vi "Inhibit Bus B.vi"(8 "error in (no error)":errorcluster, 10 "Inhibit Bus B?":bool, 11 "1553 Component in":refnum<class "1553 Component.lvclass">) -> (0 "error out":errorcluster)   [LabVIEW 2020, in "BCI-1553 API.lvlib" / "1553 Component.lvclass"]
doc: "Inhibit the operation of Bus B for this component."
uses:
  1553 Component.lvclass
  1553 Component.lvclass/1553 Component.ctl
  Dependencies/FPGA Interface/FPGA Interface.lvclass
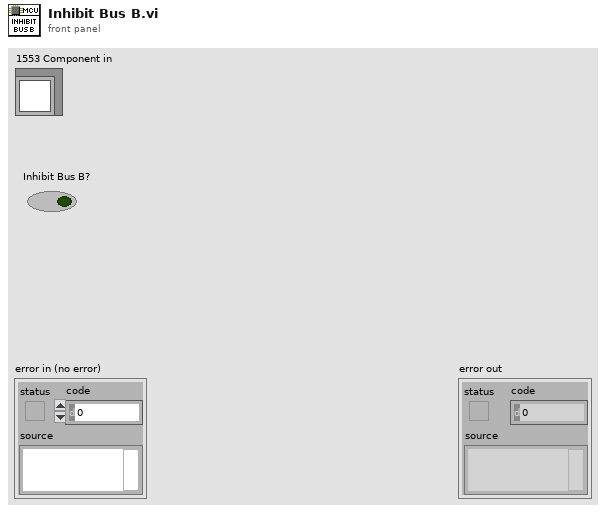
[diagram p1: front panel]
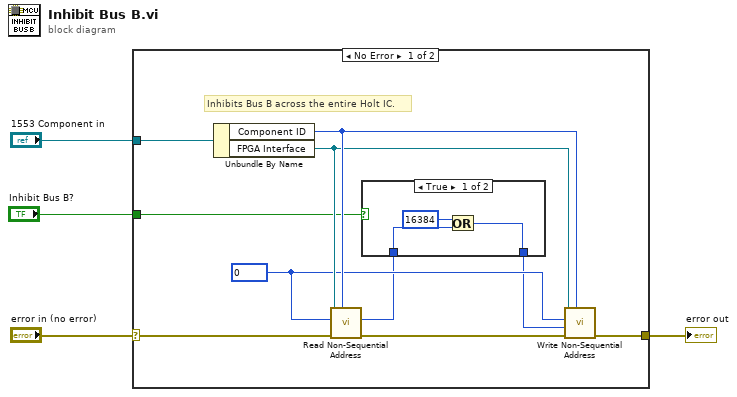
[diagram p0: block diagram]
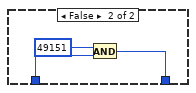
[diagram p2: hidden frame]
diagram:
  n1 = case shown="No Error" "error in (no error)" {
    selector: "error in (no error)" -> [w9 w21]
    tunnel: [w8 w21] -> w3
    tunnel: "1553 Component in" -> [w14 _]
    tunnel: "Inhibit Bus B?" -> [w6 _]
    frame No Error {
      w10 = u16 0 ("Address")
      # "Inhibits Bus B across the entire Holt IC."
      n2 = Unbundle By Name(w14) -> ("Component ID"=w13:u8, "FPGA Interface"=w12:refnum<class "FPGA Interface.lvclass">)
      n3 = call-dynamic "Read Non-Sequential Address.vi"("Target IC (1-8)"=w13, "error in (no error)"=w9, "Address"=w10, "FPGA Interface in"=w12) -> ("error out"=w11:errorcluster, "Data"=w7:u16)  [unwired: 6 in]
      n4 = case shown="True" w6 {
        tunnel: w7 -> [w17 w20]
        tunnel: [w15 w18] -> w5
        frame True {
          n5 = Or(x=u16 16384 ("Address"), y=w17) -> (x .or. y?=w15:u16)
        }
        frame False {
          n6 = And(x=u16 49151 ("Address"), y=w20) -> (x .and. y?=w18:u16)
        }
      }
      n7 = call-dynamic "Write Non-Sequential Address.vi"("Target IC (1-8)"=w13, "error in (no error)"=w11, "Data"=w5, "Address"=w10, "FPGA Interface in"=w12) -> ("error out"=w8:errorcluster)  [unwired: 6 in]
    }
    frame Error {
    }
  }
  "error out" <- w3
